vi "ADQ_bloques.vi"() -> ()   [LabVIEW 2011]
uses:
  <vilib>/DAQmx/create/channels.llb/DAQmx Create Channel (AI-Voltage-Basic).vi
  <vilib>/DAQmx/configure/timing.llb/DAQmx Timing (Sample Clock).vi
  <vilib>/DAQmx/read.llb/DAQmx Read (Analog 1D Wfm NChan NSamp).vi
panel:
  out "data 2":waveform(dbl)[](array[waveform])=[{"t0"=timestamp(3635177397.0058413 s since 1904-01-01), "dt"=0.001, "Y"=[5.2603025874275176, 5.2603025874275176, 5.26411869776388, 5.257758513869942, 5.261574624206305, 5.2653907345426685, 5.25903055064873, 5.257758513869942, 5.261574624206305, 5.2603025874275176, 5.255214440312367, 5.26411869776388, 5.2603025874275176, 5.25903055064873, 5.2603025874275176, 5.2603025874275176, 5.256486477091155, 5.26411869776388, 5.2653907345426685, 5.256486477091155, 5.2603025874275176, 5.261574624206305, 5.261574624206305, 5.255214440312367, 5.26411869776388, 5.256486477091155, 5.255214440312367, 5.26411869776388, 5.256486477091155, 5.25903055064873, 5.262846660985093, 5.257758513869942, 5.261574624206305, 5.267934808100244, 5.257758513869942, 5.2603025874275176, 5.2603025874275176, 5.261574624206305, 5.2603025874275176, 5.262846660985093, 5.257758513869942, 5.25903055064873, 5.25903055064873, 5.26411869776388, 5.2603025874275176, 5.261574624206305, 5.25903055064873, 5.2603025874275176, 5.2603025874275176, 5.274294991994182, 5.2603025874275176, 5.262846660985093, 5.256486477091155, 5.2603025874275176, 5.25903055064873, 5.25903055064873, 5.262846660985093, 5.2653907345426685, 5.257758513869942, 5.261574624206305, 5.261574624206305, 5.256486477091155, 5.2653907345426685, 5.261574624206305, 5.256486477091155, 5.25903055064873, 5.2603025874275176, 5.256486477091155, 5.262846660985093, 5.25903055064873, 5.25903055064873, 5.261574624206305, 5.262846660985093, 5.256486477091155, 5.2603025874275176, 5.262846660985093, 5.261574624206305, 5.2603025874275176, 5.255214440312367, 5.25903055064873, 5.261574624206305, 5.25903055064873, 5.2603025874275176, 5.262846660985093, 5.253942403533579, 5.25903055064873, 5.25903055064873, 5.257758513869942, 5.261574624206305, 5.25903055064873, 5.2603025874275176, 5.25903055064873, 5.262846660985093, 5.25903055064873, 5.255214440312367, 5.25903055064873, 5.25903055064873, 5.255214440312367, 5.2653907345426685, 5.257758513869942], "attributes"=variant("NI_ChannelName"=variant(string "Dev1/ai0"), "NI_UnitDescription"=variant(string "Volts"))}, {"t0"=timestamp(3635177397.005862 s since 1904-01-01), "dt"=0.001, "Y"=[2.4992449746830774, 2.49415742921149, 2.4967012019472836, 2.5005168610509743, 2.49415742921149, 2.4954293155793867, 2.5005168610509743, 2.4979730883151805, 2.4967012019472836, 2.5005168610509743, 2.4928855428435934, 2.4967012019472836, 2.4967012019472836, 2.4967012019472836, 2.4967012019472836, 2.4992449746830774, 2.4954293155793867, 2.4928855428435934, 2.4992449746830774, 2.4967012019472836, 2.4916136564756965, 2.4954293155793867, 2.4967012019472836, 2.4928855428435934, 2.4992449746830774, 2.4992449746830774, 2.49415742921149, 2.4992449746830774, 2.4967012019472836, 2.4928855428435934, 2.4967012019472836, 2.4967012019472836, 2.4928855428435934, 2.4992449746830774, 2.4954293155793867, 2.4928855428435934, 2.4967012019472836, 2.4967012019472836, 2.4928855428435934, 2.4992449746830774, 2.4967012019472836, 2.4954293155793867, 2.4967012019472836, 2.4967012019472836, 2.49415742921149, 2.4992449746830774, 2.4954293155793867, 2.49415742921149, 2.4954293155793867, 2.4979730883151805, 2.4928855428435934, 2.4992449746830774, 2.4967012019472836, 2.4928855428435934, 2.4967012019472836, 2.4954293155793867, 2.4928855428435934, 2.4992449746830774, 2.4967012019472836, 2.4954293155793867, 2.4992449746830774, 2.4967012019472836, 2.49415742921149, 2.4992449746830774, 2.4967012019472836, 2.4967012019472836, 2.4992449746830774, 2.4928855428435934, 2.4967012019472836, 2.4967012019472836, 2.4928855428435934, 2.4992449746830774, 2.5005168610509743, 2.4928855428435934, 2.4967012019472836, 2.4967012019472836, 2.4928855428435934, 2.5005168610509743, 2.4967012019472836, 2.4928855428435934, 2.4954293155793867, 2.4967012019472836, 2.4928855428435934, 2.4992449746830774, 2.5005168610509743, 2.4928855428435934, 2.4954293155793867, 2.4967012019472836, 2.4967012019472836, 2.4967012019472836, 2.5005168610509743, 2.4928855428435934, 2.4954293155793867, 2.4979730883151805, 2.4954293155793867, 2.4954293155793867, 2.4992449746830774, 2.4967012019472836, 2.4928855428435934, 2.4992449746830774], "attributes"=variant("NI_ChannelName"=variant(string "Dev1/ai1"), "NI_UnitDescription"=variant(string "Volts"))}]
  out "Waveform Chart":waveform(dbl)[](graph)=[{"t0"=timestamp(3635177397.0058413 s since 1904-01-01), "dt"=0.001, "Y"=[5.2603025874275176, 5.2603025874275176, 5.26411869776388, 5.257758513869942, 5.261574624206305, 5.2653907345426685, 5.25903055064873, 5.257758513869942, 5.261574624206305, 5.2603025874275176, 5.255214440312367, 5.26411869776388, 5.2603025874275176, 5.25903055064873, 5.2603025874275176, 5.2603025874275176, 5.256486477091155, 5.26411869776388, 5.2653907345426685, 5.256486477091155, 5.2603025874275176, 5.261574624206305, 5.261574624206305, 5.255214440312367, 5.26411869776388, 5.256486477091155, 5.255214440312367, 5.26411869776388, 5.256486477091155, 5.25903055064873, 5.262846660985093, 5.257758513869942, 5.261574624206305, 5.267934808100244, 5.257758513869942, 5.2603025874275176, 5.2603025874275176, 5.261574624206305, 5.2603025874275176, 5.262846660985093, 5.257758513869942, 5.25903055064873, 5.25903055064873, 5.26411869776388, 5.2603025874275176, 5.261574624206305, 5.25903055064873, 5.2603025874275176, 5.2603025874275176, 5.274294991994182, 5.2603025874275176, 5.262846660985093, 5.256486477091155, 5.2603025874275176, 5.25903055064873, 5.25903055064873, 5.262846660985093, 5.2653907345426685, 5.257758513869942, 5.261574624206305, 5.261574624206305, 5.256486477091155, 5.2653907345426685, 5.261574624206305, 5.256486477091155, 5.25903055064873, 5.2603025874275176, 5.256486477091155, 5.262846660985093, 5.25903055064873, 5.25903055064873, 5.261574624206305, 5.262846660985093, 5.256486477091155, 5.2603025874275176, 5.262846660985093, 5.261574624206305, 5.2603025874275176, 5.255214440312367, 5.25903055064873, 5.261574624206305, 5.25903055064873, 5.2603025874275176, 5.262846660985093, 5.253942403533579, 5.25903055064873, 5.25903055064873, 5.257758513869942, 5.261574624206305, 5.25903055064873, 5.2603025874275176, 5.25903055064873, 5.262846660985093, 5.25903055064873, 5.255214440312367, 5.25903055064873, 5.25903055064873, 5.255214440312367, 5.2653907345426685, 5.257758513869942], "attributes"=variant("NI_ChannelName"=variant(string "Dev1/ai0"), "NI_UnitDescription"=variant(string "Volts"))}, {"t0"=timestamp(3635177397.005862 s since 1904-01-01), "dt"=0.001, "Y"=[2.4992449746830774, 2.49415742921149, 2.4967012019472836, 2.5005168610509743, 2.49415742921149, 2.4954293155793867, 2.5005168610509743, 2.4979730883151805, 2.4967012019472836, 2.5005168610509743, 2.4928855428435934, 2.4967012019472836, 2.4967012019472836, 2.4967012019472836, 2.4967012019472836, 2.4992449746830774, 2.4954293155793867, 2.4928855428435934, 2.4992449746830774, 2.4967012019472836, 2.4916136564756965, 2.4954293155793867, 2.4967012019472836, 2.4928855428435934, 2.4992449746830774, 2.4992449746830774, 2.49415742921149, 2.4992449746830774, 2.4967012019472836, 2.4928855428435934, 2.4967012019472836, 2.4967012019472836, 2.4928855428435934, 2.4992449746830774, 2.4954293155793867, 2.4928855428435934, 2.4967012019472836, 2.4967012019472836, 2.4928855428435934, 2.4992449746830774, 2.4967012019472836, 2.4954293155793867, 2.4967012019472836, 2.4967012019472836, 2.49415742921149, 2.4992449746830774, 2.4954293155793867, 2.49415742921149, 2.4954293155793867, 2.4979730883151805, 2.4928855428435934, 2.4992449746830774, 2.4967012019472836, 2.4928855428435934, 2.4967012019472836, 2.4954293155793867, 2.4928855428435934, 2.4992449746830774, 2.4967012019472836, 2.4954293155793867, 2.4992449746830774, 2.4967012019472836, 2.49415742921149, 2.4992449746830774, 2.4967012019472836, 2.4967012019472836, 2.4992449746830774, 2.4928855428435934, 2.4967012019472836, 2.4967012019472836, 2.4928855428435934, 2.4992449746830774, 2.5005168610509743, 2.4928855428435934, 2.4967012019472836, 2.4967012019472836, 2.4928855428435934, 2.5005168610509743, 2.4967012019472836, 2.4928855428435934, 2.4954293155793867, 2.4967012019472836, 2.4928855428435934, 2.4992449746830774, 2.5005168610509743, 2.4928855428435934, 2.4954293155793867, 2.4967012019472836, 2.4967012019472836, 2.4967012019472836, 2.5005168610509743, 2.4928855428435934, 2.4954293155793867, 2.4979730883151805, 2.4954293155793867, 2.4954293155793867, 2.4992449746830774, 2.4967012019472836, 2.4928855428435934, 2.4992449746830774], "attributes"=variant("NI_ChannelName"=variant(string "Dev1/ai1"), "NI_UnitDescription"=variant(string "Volts"))}]
  in  "physical channels":tag="Dev1/ai0:1"
  in  "rate":dbl=1000.0 format="%0.2f"
  in  "stop":bool
  in  "number of samples per channel":i32=100
  in  "minimum value":dbl=-6.0 format="%0.2f"
  in  "maximum value":dbl=6.0 format="%0.2f"
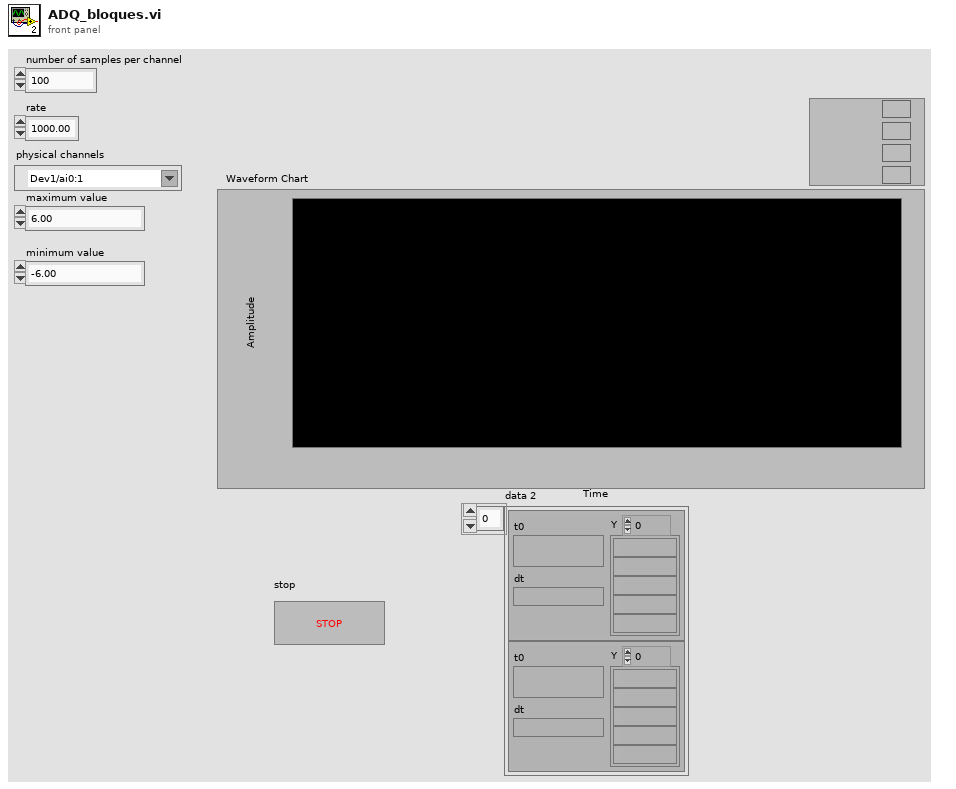
[diagram p1: front panel]
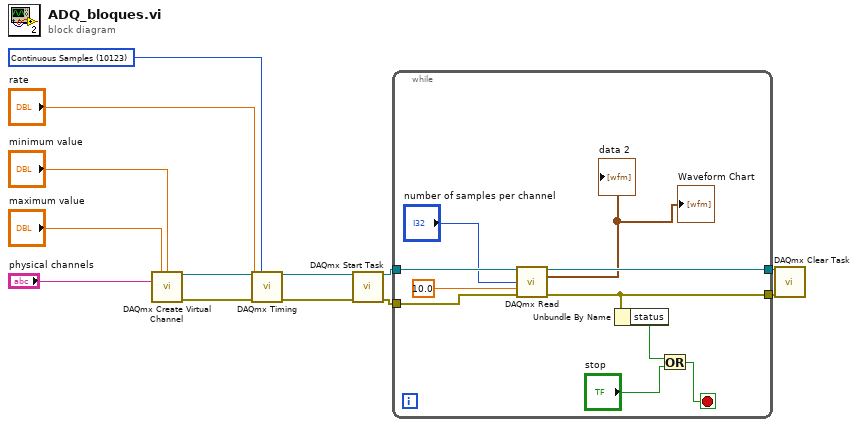
[diagram p0: block diagram]
diagram:
  w5 = 10123 items=["Finite Samples"=10178, "Continuous Samples"=10123, "Hardware Timed Single Point"=12522] ("sample mode")
  n1 = call-poly <vilib>:"DAQmx Create Virtual Channel.vi"("maximum value"="maximum value", "minimum value"="minimum value", "physical channels"="physical channels") -> ("task out"=w11:refnum<k21>, "error out"=w10:errorcluster)  [unwired: 11 in]
  n2 = call-poly <vilib>:"DAQmx Timing.vi"("task/channels in"=w11, "sample mode"=w5, "rate"="rate", "error in"=w10) -> ("task out"=w9:refnum<k21>, "error out"=w8:errorcluster)  [unwired: 10 in]
  n3 = call <vilib>:"DAQmx Start Task.vi"("task/channels in"=w9, "error in"=w8) -> ("task out"=w7:refnum<k21>, "error out"=w6:errorcluster)  [unwired: 12 in]
  n4 = while {
    tunnel: w7 -> [w23]
    tunnel: w6 -> [w22]
    tunnel: [w19] -> w2
    tunnel: [w18] -> w1
    stop <- w15 stop-if-true
    n5 = call-poly <vilib>:"DAQmx Read.vi"("task/channels in"=w23, "number of samples per channel"="number of samples per channel", "timeout"=10.0, "error in"=w22) -> ("task out"=w18:refnum<k21>, "data"=→"Waveform Chart" →"data 2":waveform(dbl)[], "error out"=w19:errorcluster)  [unwired: 9 in]
    n6 = Unbundle By Name(w19) -> ("status"=w17:bool)
    n7 = Or(x=w17, y="stop") -> (x .or. y?=w15:bool)
  }
  n8 = call <vilib>:"DAQmx Clear Task.vi"("task in"=w1, "error in"=w2) -> ()  [unwired: 13 in, 1 out]
